vi "Cycle.vi"(8 "error in (no error)":errorcluster, 11 "TwoAfcEye In":refnum<class "TwoAfcEye.lvclass">) -> (0 "error out":errorcluster, 3 "TwoAfcEye Out":refnum<class "TwoAfcEye.lvclass">)   [LabVIEW 2014, in "TwoAfcEye.lvclass"]
uses:
  TwoAfcEye.lvclass
  Trial Based Experiment Statechart/MatlabExperiment/MatlabExperiment.lvclass
panel:
  out "ExperimentStats":T1
  in  "FixationRadius":dbl=34.0
  in  "RewardAmount":dbl=50.0
  out "Timeouts":T2={"Intertrial"=1500.0, "AcquireFixation"=4000.0, "HoldFixation"=300.0, "DelayPeriod"=2000.0, "ResponsePeriod"=0.0}
  in  "Eye Params":dbl[](array[numeric])
  out "XY Graph":cluster{"horizontal":dbl[], "vertical":dbl[]}[](graph)
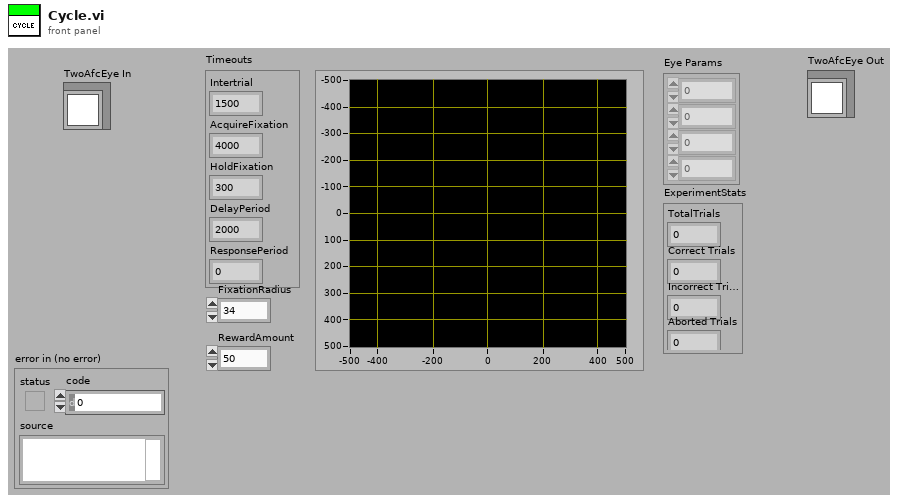
[diagram p1: front panel]
types:
  T1 = cluster{"TotalTrials":dbl, "Correct Trials":dbl, "Incorrect Trials":dbl, "Aborted Trials":dbl}
  T2 = cluster{"Intertrial":dbl, "AcquireFixation":dbl, "HoldFixation":dbl, "DelayPeriod":dbl, "ResponsePeriod":dbl}
  T3 = cluster{"TotalTrials":u32, "Correct Trials":u32, "Incorrect Trials":u32, "Aborted Trials":u32}
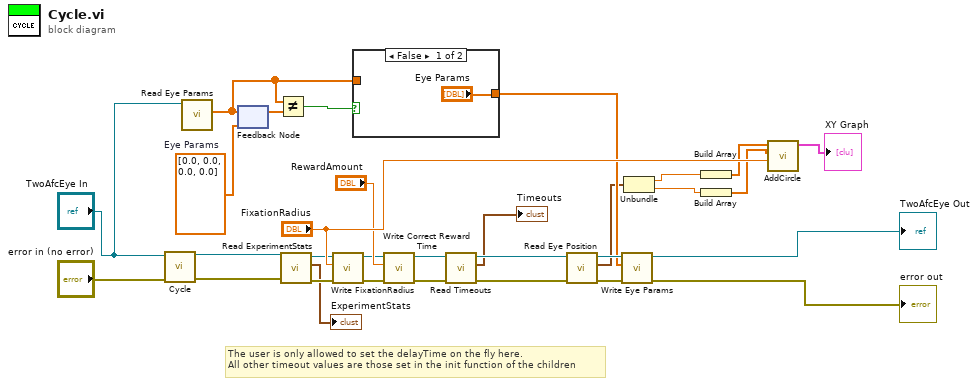
[diagram p0: block diagram]
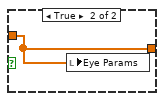
[diagram p2: hidden frame]
diagram:
  w14 = dbl[] [0.0, 0.0, 0.0, 0.0]  # Eye Params
  # "The user is only allowed to set the delayTime on the fly here. \nAll other timeout values are those set in the init function of the children"
  n1 = call-parent "Cycle.vi"("error in (no error)"="error in (no error)", "MatlabExperiment In"="TwoAfcEye In") -> ("error out"=w7:errorcluster, "MatlabExperiment Out"=w8:refnum<class "TwoAfcEye.lvclass">)  [unwired: 8 in]
  n2 = call-dynamic "Read Eye Params.vi"("TrialBasedExperiment in"="TwoAfcEye In") -> ("Eye Params"=w13:dbl[])  [unwired: 8 in, 2 out]
  n3 = feedback #1(w14) -> (w16:dbl[])
  n4 = feedback-in #1(w13) -> ()
  n5 = Not Equal?(x=w13, y=w16) -> (x != y?=w15:bool)
  n6 = call-dynamic "Read ExperimentStats.vi"("error in (no error)"=w7, "TrialBasedExperiment in"=w8) -> ("error out"=w23:errorcluster, "ExperimentStats"=→"ExperimentStats":T3, "TrialBasedExperiment out"=w24:refnum<class "TwoAfcEye.lvclass">)  [unwired: 7 in]
  n7 = call-dynamic "Write FixationRadius.vi"("error in (no error)"=w23, "FixationRadius"="FixationRadius", "MatlabExperiment in"=w24) -> ("error out"=w20:errorcluster, "MatlabExperiment out"=w21:refnum<class "TwoAfcEye.lvclass">)  [unwired: 7 in]
  n8 = case shown="False" w15 {
    tunnel: ["Eye Params" w33] -> w10
    tunnel: w13 -> [_ w33]
    frame False {
    }
    frame True {
      n9 = local write "Eye Params"(w33) -> ()
    }
  }
  n10 = call-dynamic "Write Correct Reward Time.vi"("error in (no error)"=w20, "Correct Reward Time"="RewardAmount", "MatlabExperiment in"=w21) -> ("error out"=w18:errorcluster, "MatlabExperiment out"=w19:refnum<class "TwoAfcEye.lvclass">)  [unwired: 7 in]
  n11 = call-dynamic "Read Timeouts.vi"("error in (no error)"=w18, "TrialBasedExperiment in"=w19) -> ("error out"=w2:errorcluster, "Timeouts"=→"Timeouts":T2, "TrialBasedExperiment out"=w3:refnum<class "TwoAfcEye.lvclass">)  [unwired: 7 in]
  n12 = call-dynamic "Read Eye Position.vi"("error in (no error)"=w2, "TrialBasedExperiment in"=w3) -> ("error out"=w11:errorcluster, "Eye Position"=w9:cluster{"Horizontal":dbl, "Vertical":dbl}, "TrialBasedExperiment out"=w12:refnum<class "TwoAfcEye.lvclass">)  [unwired: 7 in]
  n13 = call-dynamic "Write Eye Params.vi"("error in (no error)"=w11, "Eye Params"=w10, "TrialBasedExperiment in"=w12) -> ("error out"=→"error out":errorcluster, "TrialBasedExperiment out"=→"TwoAfcEye Out":refnum<class "TwoAfcEye.lvclass">)  [unwired: 7 in]
  n14 = Unbundle(w9) -> ("Horizontal"=w25:dbl, "Vertical"=w26:dbl)
  n15 = Build Array(w25) -> (w27:dbl[])
  n16 = Build Array(w26) -> (w28:dbl[])
  n17 = call "AddCircle.vi"("radius"="FixationRadius", "vertical"=w28, "horizontal"=w27) -> ("output"=→"XY Graph":cluster{"horizontal":dbl[], "vertical":dbl[]}[])  [unwired: 8 in]
